vi "Keith 7001 Initialize.vi"(0 "GPIB address in":string, 1 "ID query":bool, 2 "reset":bool, 3 "error in":T1, 4 "error query":bool) -> (5 "GPIB address out":string, 6 "error out":T1)   [LabVIEW 2019]
doc: "This VI loads the addressing information about the instrument into the Open VXI Instrument VI and returns the instrument ID. You can optionally reset the instrument by setting the front panel reset control. You must run this VI before using any of the instrument driver VIs for this instrument."
panel:
  # "yes\nno"
  # "yes\nno"
  # "yes\nno"
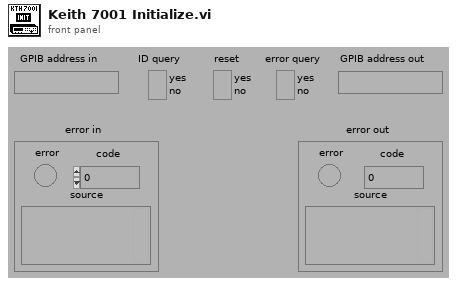
[diagram p1: front panel]
types:
  T1 = cluster{"error":bool, "code":i32, "source":string}
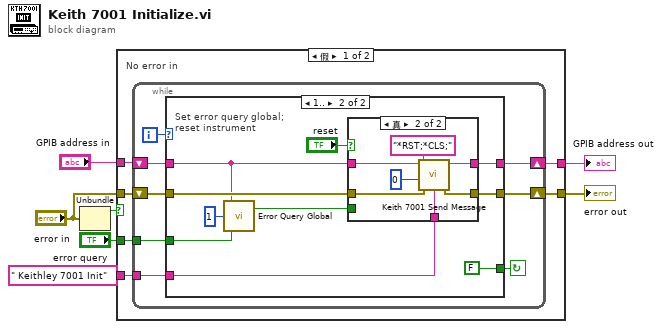
[diagram p0: block diagram]
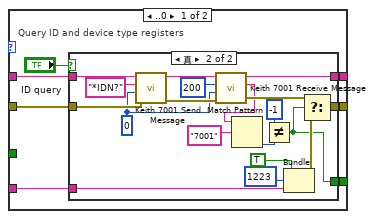
[diagram p2: hidden frame]
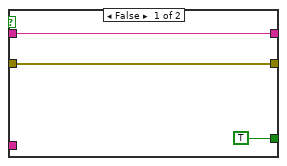
[diagram p3: hidden frame]
diagram:
  n1 = Unbundle("error in") -> ("error"=w6:bool)  [unwired: 2 out]
  n2 = case shown="假" w6 {
    tunnel: "error in" -> [w13 w71]
    tunnel: " Keithley 7001 Init" -> [w12 _]
    tunnel: [w11 w71] -> w1
    tunnel: [w10 "-1"] -> w3
    tunnel: "error query" -> [w9 _]
    tunnel: "GPIB address in" -> [w8 _]
    frame False {
      # "No error in"
      n3 = while {
        tunnel: w9 -> [w16]
        tunnel: w12 -> [w17]
        shift-left: w8 -> [w18]
        shift-right: [w14] -> w10
        shift-left: w13 -> [w21]
        shift-right: [w15] -> w11
        i -> [w19]
        stop <- w20 continue-if-true
        n4 = case shown="1.." w19 {
          tunnel: w21 -> [w27 w59]
          tunnel: [w24 w58] -> w15
          tunnel: [w23 FALSE] -> w20
          tunnel: [w25 w60] -> w14
          tunnel: w18 -> [w26 w54]
          tunnel: w17 -> [w28 w55]
          tunnel: w16 -> [_ w52]
          frame ..0 {
            # "Query ID and device type registers"
            n5 = case shown="真" "ID query" {
              tunnel: [w30 w46] -> w24
              tunnel: w27 -> [w30 w40]
              tunnel: [w31 w38] -> w25
              tunnel: w26 -> [w31 w44]
              tunnel: w28 -> [_ w45]
              tunnel: [TRUE w33] -> w23
              frame False {
              }
              frame True {
                w37 = 0
                n6 = call "Keith 7001 Send Message.vi"("address string"=w44, "write buffer"="*IDN?", "write mode (set END:0)"=w37, "error in"=w40) -> ("address out"=w43:string, "error out"=w39:T1)  [unwired: 2 in, 2 out]
                n7 = call "Keith 7001 Receive Message.vi"("address string"=w43, "byte count"=200, "read mode"=w37, "error in"=w39) -> ("address out"=w38:string, "read buffer"=w35:string, "error out"=w50:T1)  [unwired: 2 in, 1 out]
                n8 = Match Pattern(string=w35, regular expression="7001") -> (offset past match=w34:i32)  [unwired: 1 in, 3 out]
                n9 = Not Equal?(x=-1, y=w34) -> (x != y?=w33:bool)
                n10 = Bundle(TRUE, 1223, w45) -> (w49:errorcluster)  [unwired: 1 in]
                n11 = Select(t=w50, s=w33, f=w49) -> (s? t:f=w46:T1)
              }
            }
          }
          frame 1.. {
            # "Set error query global;\nreset instrument"
            n12 = call "Error Query Global.vi"("new error query setting"=w52, "mode (0:read value)"=u16 1, "GPIB address"=w54) -> ("address already present?"=w51:bool)  [unwired: 1 out]
            n13 = case shown="真" "reset" {
              tunnel: [w61 w67] -> w60
              tunnel: w54 -> [w61 w66]
              tunnel: w59 -> [w62 w65]
              tunnel: [w62 w64] -> w58
              tunnel: w55 -> [_ w63]
              tunnel: w51 -> [_ _]
              frame False {
              }
              frame True {
                n14 = call "Keith 7001 Send Message.vi"("address string"=w66, "write buffer"="*RST;*CLS;", "source"=w63, "write mode (set END:0)"=0, "error in"=w65) -> ("address out"=w67:string, "error out"=w64:T1)  [unwired: 1 in, 2 out]
              }
            }
          }
        }
      }
    }
    frame True {
      # "Error in"
    }
  }
  "GPIB address out" <- w3
  "error out" <- w1
